vi "v2.12.vi"() -> ()   [LabVIEW 2018]
uses:
  <vilib>/DAQmx/read.llb/DAQmx Read (Analog 1D DBL NChan 1Samp).vi
  <vilib>/DAQmx/create/channels.llb/DAQmx Create Channel (AI-Temperature-Thermocouple).vi
  <vilib>/DAQmx/configure/timing.llb/DAQmx Timing (Sample Clock).vi
  <vilib>/DAQmx/miscellaneous.llb/DAQmx Fill In Error Info.vi
panel:
  out "Waveform Chart":dbl(graph)
  out "Array":dbl[][](array[numeric])
  in  "Noise":dbl(knob) scale=0.0..5.0
  in  "Flow Controls":dbl(slide) min=-100.0 max=100.0 scale=-100.0..100.0
  out "Status":T1(ring)
  out "Live Display":dbl[](array[numeric])
  in  "Stop":bool
  in  "OK Button":bool
  in  "DAQ Properties":cluster{"Sample Rate":dbl}
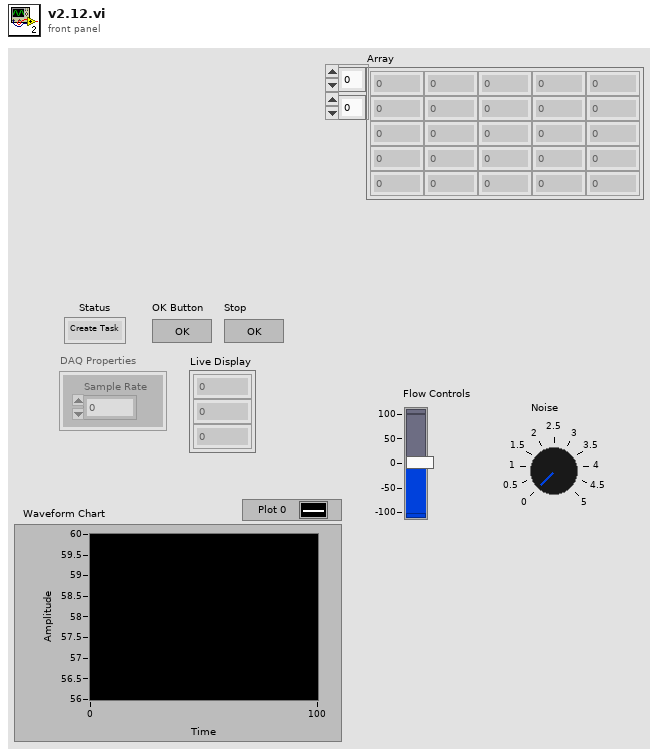
[diagram p1: front panel]
types:
  T1 = enum16{"Create Task", "Change Settings", "Check Settings", "Read Data", "End Task"}
  T2 = enum8{"Enabled", "Disabled", "Disabled and Grayed Out"}
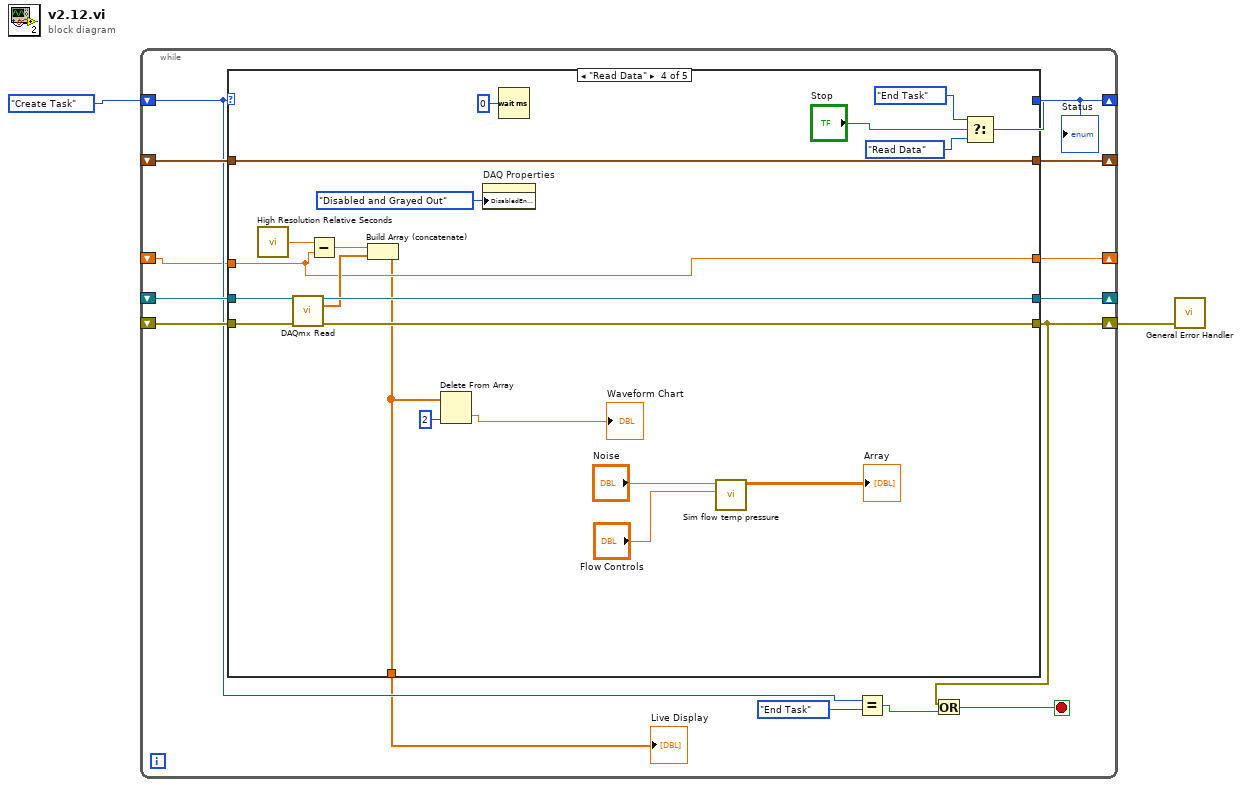
[diagram p0: block diagram]
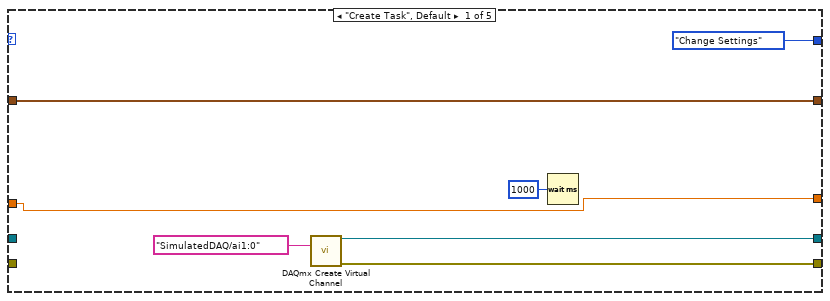
[diagram p2: hidden frame]
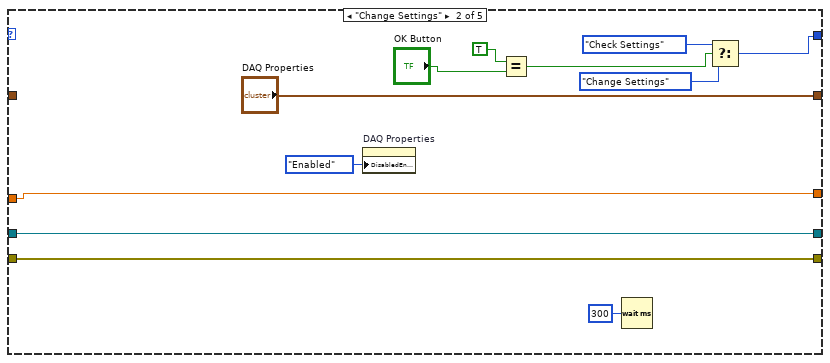
[diagram p3: hidden frame]
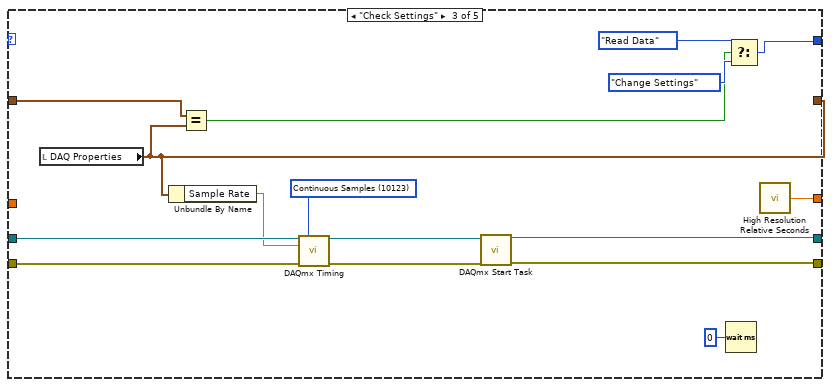
[diagram p4: hidden frame]
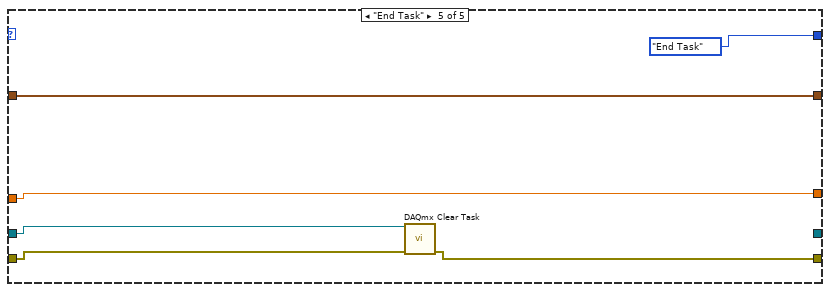
[diagram p5: hidden frame]
diagram:
  n1 = while {
    shift-right: [w11] -> _
    shift-left: T1."Create Task" -> [w6]
    shift-right: [w16] -> _
    shift-left: _ -> [w14]
    shift-right: [w10] -> w1
    shift-left: _ -> [w13]
    shift-right: [w15] -> _
    shift-left: _ -> [w12]
    shift-right: [w5] -> _
    shift-left: _ -> [w4]
    stop <- w9 stop-if-true
    n2 = case shown="\"Read Data\"" w6 {
      tunnel: [w23 w35 w40 w69 _] -> w16
      tunnel: [w22 w34 w39 w68 w78] -> w10
      tunnel: [T1."Change Settings" w28 w47 w66 T1."End Task"] -> w11
      tunnel: [w19 "DAQ Properties" w43 w70 w77] -> w15
      tunnel: w14 -> [_ w35 w46 w72 w75]
      tunnel: w13 -> [_ w34 w45 w71 w74]
      tunnel: w12 -> [w19 _ w51 w70 w77]
      tunnel: [w17 w25 w36 w59 w73] -> w5
      tunnel: w4 -> [w17 w25 _ w59 w73]
      tunnel: [_ _ _ w54 _] -> w3
      frame "Create Task", Default {
        n3 = call-poly <vilib>:"DAQmx Create Virtual Channel.vi"("physical channels"=tag "SimulatedDAQ/ai1:0") -> ("task out"=w23:refnum<k21>, "error out"=w22:errorcluster)  [unwired: 13 in]
        n4 = Wait (ms)(milliseconds to wait=u32 1000) -> ()  [unwired: 1 out]
      }
      frame "Change Settings" {
        n5 = property on="DAQ Properties" class="Clust (strict)"("DisabledEnum"=T2."Enabled" ("Disabled")) -> ()  [unwired: 2 in, 2 out]
        n6 = Equal?(x=TRUE, y="OK Button") -> (x = y?=w30:bool)
        n7 = Wait (ms)(milliseconds to wait=u32 300) -> ()  [unwired: 1 out]
        n8 = Select(t=T1."Check Settings", s=w30, f=T1."Change Settings") -> (s? t:f=w28:T1)
      }
      frame "Check Settings" {
        w37 = 10123 items=["Finite Samples"=10178, "Continuous Samples"=10123, "Hardware Timed Single Point"=12522] ("sample mode")
        n9 = local read "DAQ Properties"() -> (w43:cluster{"Sample Rate":dbl})
        n10 = Unbundle By Name(w43) -> ("Sample Rate"=w44:dbl)
        n11 = Equal?(x=w51, y=w43) -> (x = y?=w38:bool)
        n12 = call-poly <vilib>:"DAQmx Timing.vi"("task/channels in"=w46, "sample mode"=w37, "rate"=w44, "error in"=w45) -> ("task out"=w42:refnum<k21>, "error out"=w41:errorcluster)  [unwired: 10 in]
        n13 = call <vilib>:"DAQmx Start Task.vi"("task/channels in"=w42, "error in"=w41) -> ("task out"=w40:refnum<k21>, "error out"=w39:errorcluster)  [unwired: 12 in]
        n14 = Wait (ms)(milliseconds to wait=u32 0) -> ()  [unwired: 1 out]
        n15 = Select(t=T1."Read Data", s=w38, f=T1."Change Settings") -> (s? t:f=w47:T1)
        n16 = call <vilib>:"High Resolution Relative Seconds.vi"() -> ("relative seconds"=w36:dbl)
      }
      frame "Read Data" {
        n17 = call <vilib>:"High Resolution Relative Seconds.vi"() -> ("relative seconds"=w62:dbl)
        n18 = call-poly <vilib>:"DAQmx Read.vi"("task/channels in"=w72, "error in"=w71) -> ("task out"=w69:refnum<k21>, "data"=w61:dbl[], "error out"=w68:errorcluster)  [unwired: 11 in]
        n19 = Subtract(x=w62, y=w59) -> (x-y=w60:dbl)
        n20 = Build Array (concatenate)(w60, w61) -> (w54:dbl[])
        n21 = Delete From Array(array=w54, index=2) -> (deleted portion=→"Waveform Chart":dbl)  [unwired: 1 in, 1 out]
        n22 = property on="DAQ Properties" class="Clust (strict)"("DisabledEnum"=T2."Disabled and Grayed Out" ("Disabled")) -> ()  [unwired: 2 in, 2 out]
        n23 = Wait (ms)(milliseconds to wait=u32 0) -> ()  [unwired: 1 out]
        n24 = call "Sim flow temp pressure.vi"("Offset"="Flow Controls", "Spectral Amplitude"="Noise") -> ("Array"=→"Array":dbl[][])  [unwired: 9 in]
        n25 = Select(t=T1."End Task", s="Stop", f=T1."Read Data") -> (s? t:f=w66:T1)
      }
      frame "End Task" {
        n26 = call <vilib>:"DAQmx Clear Task.vi"("task in"=w75, "error in"=w74) -> ("error out"=w78:errorcluster)  [unwired: 13 in]
      }
    }
    "Live Display" <- w3
    "Status" <- w11
    n27 = Equal?(x=w6, y=T1."End Task") -> (x = y?=w7:bool)
    n28 = Or(x=w10, y=w7) -> (x .or. y?=w9:bool)
  }
  n29 = call <vilib>:"General Error Handler.vi"("error in (no error)"=w1) -> ()  [unwired: 10 in, 5 out]
